vi "Testing.vi"() -> ()   [LabVIEW 2025]
uses:
  <vilib>/measure/madcrms.llb/Basic Averaged DC-RMS for N Chan.vi
  <vilib>/measure/NI_MAPro.lvlib
panel:
  out "Mains Request":sgl
  out "Loop":i32
  out "Bus Current Load Demand":dbl
  out "Bus Voltage RMS/100":dbl
  out "Bus Current Demand to SM":dynamicdata(graph)
  out "All Output Graphs":dynamicdata(graph)
  out "Battery Charge Sw":bool
  out "Battery Discharge Sw":bool
  out "LoadSw3":bool
  out "LoadSw2":bool
  out "LoadSw1":bool
  out "SM PV Current":dbl
  out "SM Wind Current":dbl
  in  "Manual Control\nPV % of Max.":dbl(knob) scale=0.0..100.0
  in  "Manual Control\nWind % of Max.":dbl(knob) scale=0.0..100.0
  in  "Load 3":bool
  in  "Load 2":bool
  in  "Load 1":bool
  out "Bus Current (rms)":dynamicdata(graph)
  out "Bus Voltage (rms)":dynamicdata(graph)
  out "Load 3":bool
  out "Load 2":bool
  out "Load 1":bool
  out "Charge Batt":bool
  out "Discharge Batt":bool
  out "Analog Input (Main Capacity 0-10V)":dynamicdata(graph)
  in  "stop":bool
  out "Voltage Dip Supply < Demand":dynamicdata(graph)
  out "240 Vrms Supply >=Demand":dynamicdata(graph)
  out "Capacity - Demand (current)":dynamicdata(graph)
  in  "Battery Charging Current":dbl
  in  "Battery Disharging Current":dbl
  in  "Load 3 Demand (current)":dbl
  in  "Load 2 Demand (current)":dbl
  in  "Load 1 Demand (current)":dbl
  out "Battery Charging Current":dynamicdata(graph)
  out "Load 3 Current":dynamicdata(graph)
  out "Load 2 Current":dynamicdata(graph)
  out "Load 1 Current":dynamicdata(graph)
  out "Battery Discharging Current (A rms)":dynamicdata(graph)
  out "Main Available Current (A rms)":dynamicdata(graph)
  out "PV Available Current (A rms)":dynamicdata(graph)
  out "Wind Available Current (A rms)":dynamicdata(graph)
  in  "Main capacity (current)":dbl
  in  "Max PV capacity (current)":dbl
  in  "Max wind capacity (current)":dbl
  out "Bus Voltage 240Vrms/100":dynamicdata(graph)
  # "Smart Meter Emulator Algorithm inputs and output status"
  # "Manual testing of Wind/PV inputs and Load calls without using the test bed  - Output graph on right - by Russel Torah - 2021"
  # "Manual Control of Load selection \nPress Load button to activate"
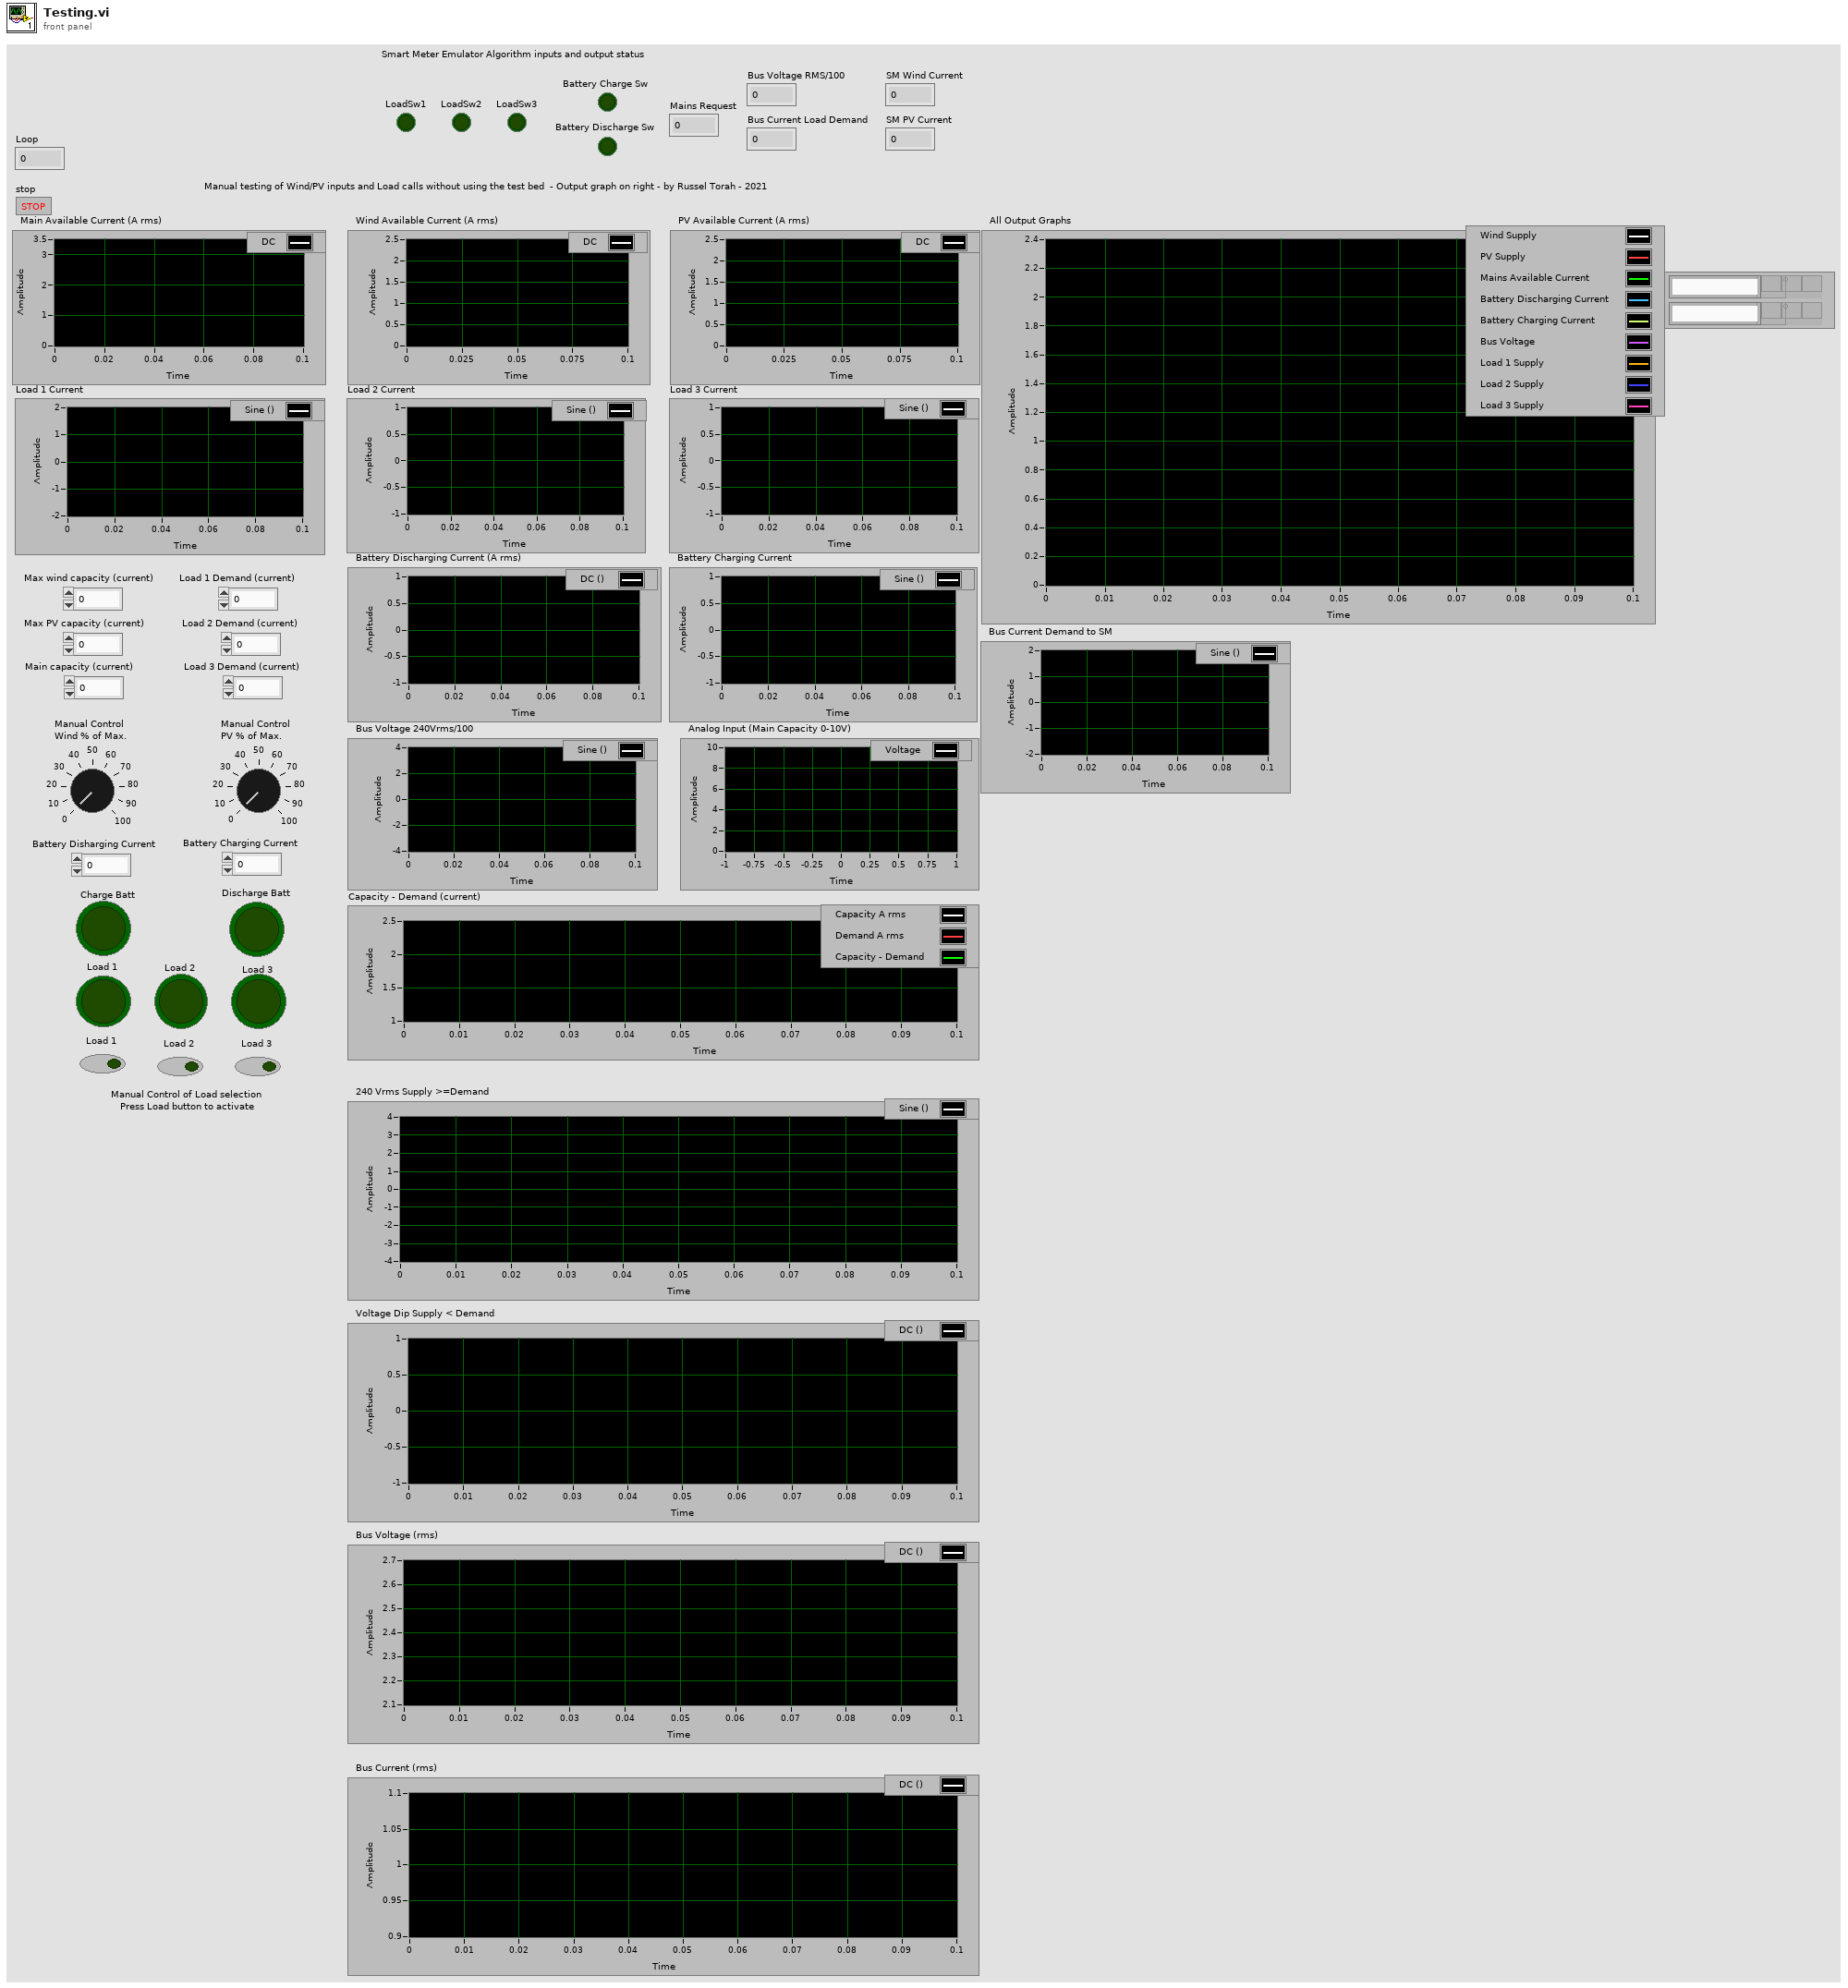
[diagram p1: front panel]
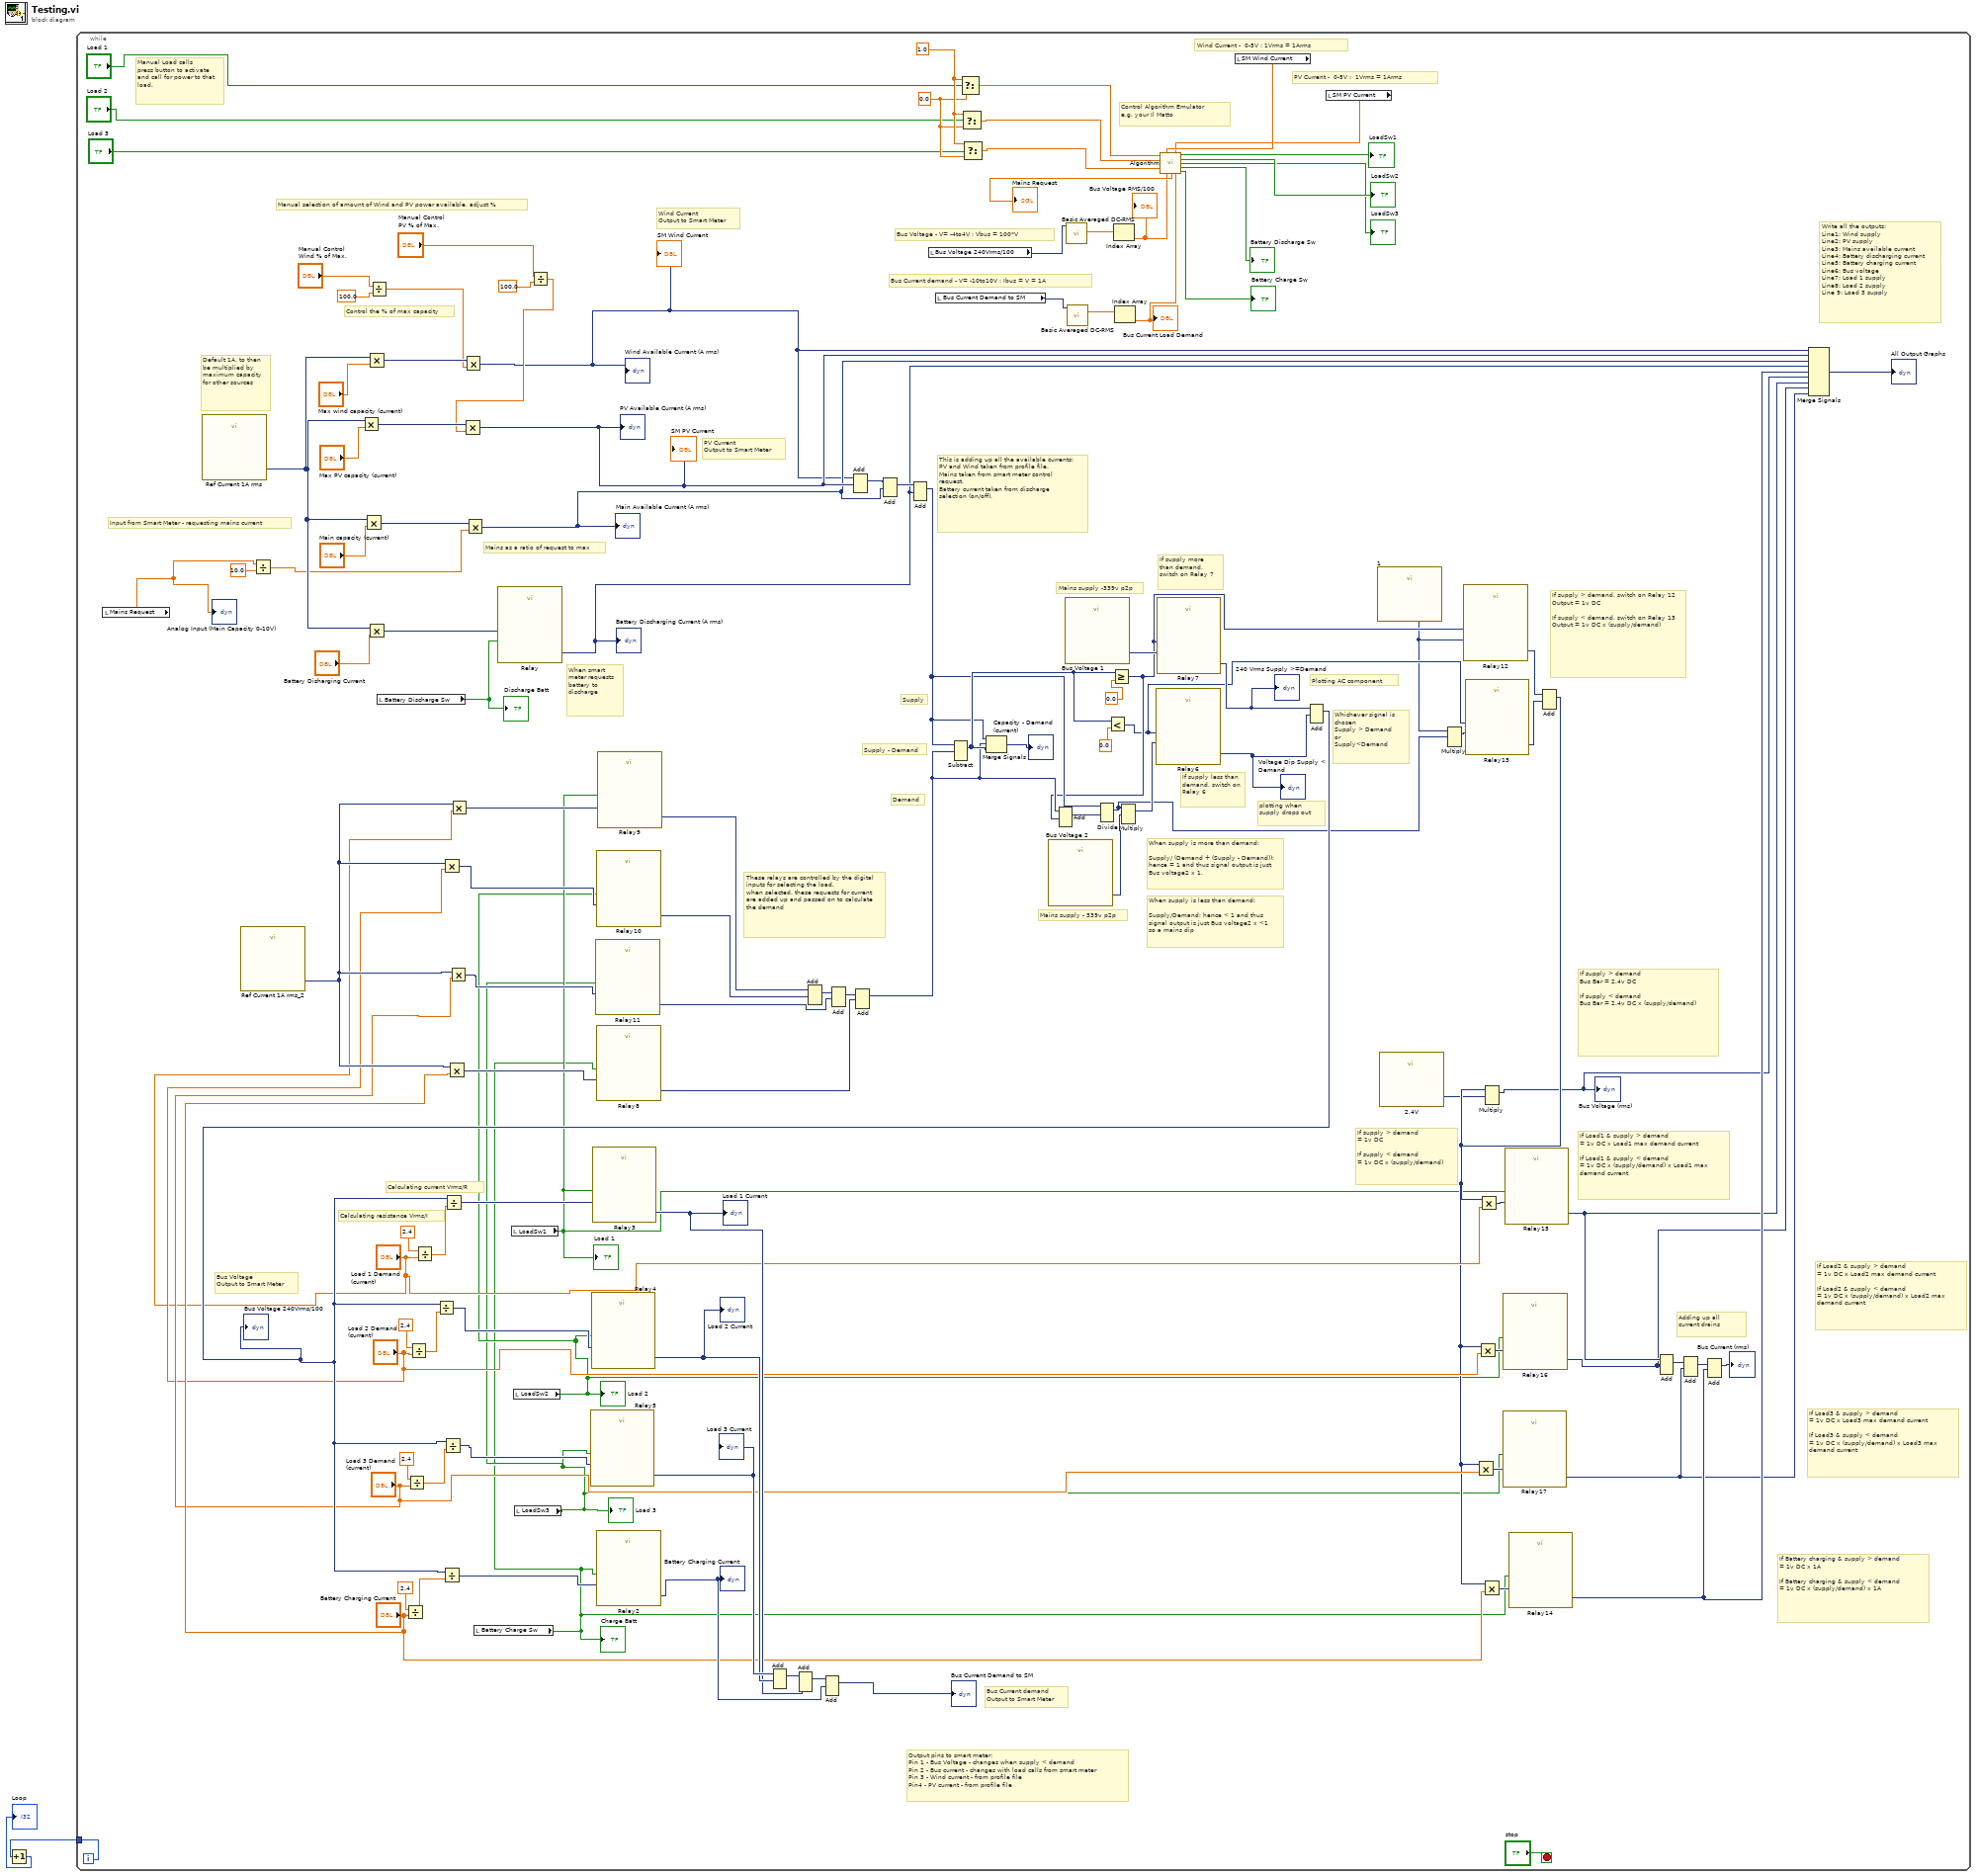
[diagram p0: block diagram]
diagram:
  n1 = while {
    tunnel: [w3] -> w2
    i -> [w3]
    stop <- "stop" stop-if-true
    w32 = 0.0 ("f")
    w33 = 1.0 ("t")
    # "Bus Current demand - V= -10to10V : Ibus = V = 1A"
    # "Bus Voltage - V= -4to4V : Vbus = 100*V"
    # "Wind Current -  0-5V : 1Vrms = 1Arms"
    # "PV Current -  0-5V :  1Vrms = 1Arms"
    # "PV Current\nOutput to Smart Meter"
    # "Wind Current\nOutput to Smart Meter"
    # "Bus Current demand\nOutput to Smart Meter"
    # "Bus Voltage\nOutput to Smart Meter"
    # "Control Algorithm Emulator\ne.g. your Il Matto"
    # "Control the % of max capacity"
    # "Manual selection of amount of Wind and PV power available, adjust %"
    # "Manual Load calls\npress button to activate and call for power to that load."
    # "Plotting AC component"
    # "plotting when supply drops out"
    # "Output pins to smart meter:\nPin 1 - Bus Voltage - changes when supply < demand\nPin 2 - Bus current - changes with load calls from smart meter\nPin 3 - Wind current - from profile file\nPin4 - PV current - from profile file"
    # "When smart meter requests battery to discharge"
    # "Mains as a ratio of request to max"
    # "Write all the outputs:\nLine1: Wind supply\nLine2: PV supply\nLine3: Mains available current\nLine4: Battery discharging current\nLine5: Battery charging current\nLine6: Bus voltage\nLine7: Load 1 supply\nLine8: Load 2 supply\nLine 9: Load 3 supply"
    # "Adding up all current drains"
    # "If Battery charging & supply > demand\n= 1v DC x 1A\n\nIf Battery charging & supply < demand\n= 1v DC x (supply/demand) x 1A"
    # "If Load3 & supply > demand\n= 1v DC x Load3 max demand current\n\nIf Load3 & supply < demand\n= 1v DC x (supply/demand) x Load3 max demand current"
    # "If Load2 & supply > demand\n= 1v DC x Load2 max demand current\n\nIf Load2 & supply < demand\n= 1v DC x (supply/demand) x Load2 max demand current"
    # "If Load1 & supply > demand\n= 1v DC x Load1 max demand current\n\nIf Load1 & supply < demand\n= 1v DC x (supply/demand) x Load1 max demand current"
    # "If supply > demand\n= 1v DC\n\nIf supply < demand\n= 1v DC x (supply/demand)"
    # "If supply > demand\nBus Bar = 2.4v DC\n\nIf supply < demand\nBus Bar = 2.4v DC x (supply/demand)"
    # "If supply > demand, switch on Relay 12\nOutput = 1v DC\n\nIf supply < demand, switch on Relay 13\nOutput = 1v DC x (supply/demand)"
    # "Whichever signal is chosen\nSupply > Demand\nor\nSupply<Demand"
    # "When supply is less than demand:\n\nSupply/Demand; hence < 1 and thus signal output is just Bus voltage2 x <1 so a mains dip"
    # "When supply is more than demand:\n\nSupply/ (Demand + (Supply - Demand)); hence = 1 and thus signal output is just Bus voltage2 x 1."
    # "Demand"
    # "Supply"
    # "If supply less than demand, switch on Relay 6"
    # "If supply more than demand, switch on Relay 7"
    # "Mains supply - 339v p2p"
    # "Mains supply -339v p2p"
    # "Supply - Demand"
    # "Calculating current Vrms/R"
    # "Calculating resistance Vrms/I"
    # "These relays are controlled by the digital inputs for selecting the load.\nwhen selected, these requests for current are added up and passed on to calculate the demand"
    # "Default 1A, to then be multiplied by maximum capacity for other sources"
    # "Input from Smart Meter - requesting mains current"
    # "This is adding up all the available currents:\nPV and Wind taken from profile file.\nMains taken from smart meter control request.\nBattery current taken from discharge selection (on/off)."
    n2 = local read "Mains Request"() -> (w15:sgl)
    "Analog Input (Main Capacity 0-10V)" <- w15
    n3 = call "Ref Current 1A rms"() -> ("DC"=w113:dynamicdata)  [unwired: 14 in, 1 out]
    n4 = call "Ref Current 1A rms_2"() -> ("DC"=w72:dynamicdata)  [unwired: 14 in, 1 out]
    n5 = Divide(x=w15, y=10.0) -> (x/y=w81:dbl)
    n6 = Multiply(x=w113, y="Max PV capacity (current)") -> (x*y=w122:dynamicdata)
    n7 = Multiply(x=w113, y="Main capacity (current)") -> (x*y=w121:dynamicdata)
    n8 = Multiply(x=w113, y="Max wind capacity (current)") -> (x*y=w123:dynamicdata)
    n9 = Multiply(x=w113, y="Battery Disharging Current") -> (x*y=w120:dynamicdata)
    n10 = Divide(x="Manual Control\nWind % of Max.", y=100.0) -> (x/y=w37:dbl)
    n11 = local read "Battery Discharge Sw"() -> (w11:bool)
    "Discharge Batt" <- w11
    n12 = Divide(x=2.4, y="Battery Charging Current") -> (x/y=w101:dbl)
    n13 = Divide(x=2.4, y="Load 3 Demand (current)") -> (x/y=w103:dbl)
    n14 = Divide(x=2.4, y="Load 2 Demand (current)") -> (x/y=w106:dbl)
    n15 = Divide(x=2.4, y="Load 1 Demand (current)") -> (x/y=w109:dbl)
    n16 = Multiply(x=w72, y="Load 2 Demand (current)") -> (x*y=w96:dynamicdata)
    n17 = Multiply(x=w72, y="Battery Charging Current") -> (x*y=w94:dynamicdata)
    n18 = Multiply(x=w72, y="Load 3 Demand (current)") -> (x*y=w95:dynamicdata)
    n19 = Multiply(x=w72, y="Load 1 Demand (current)") -> (x*y=w97:dynamicdata)
    n20 = Multiply(x=w123, y=w37) -> (x*y=w25:dynamicdata)
    "Wind Available Current (A rms)" <- w25
    "SM Wind Current" <- w25
    n21 = Multiply(x=w121, y=w81) -> (x*y=w66:dynamicdata)
    "Main Available Current (A rms)" <- w66
    n22 = local read "Battery Charge Sw"() -> (w12:bool)
    "Charge Batt" <- w12
    n23 = call "Relay"("Enable"=w11, "Signals"=w120) -> ("Result"=w65:dynamicdata)  [unwired: 8 in, 1 out]
    "Battery Discharging Current (A rms)" <- w65
    n24 = local read "LoadSw1"() -> (w21:bool)
    "Load 1" <- w21
    n25 = local read "LoadSw2"() -> (w14:bool)
    "Load 2" <- w14
    n26 = local read "LoadSw3"() -> (w13:bool)
    "Load 3" <- w13
    n27 = Divide(x="Manual Control\nPV % of Max.", y=100.0) -> (x/y=w34:dbl)
    n28 = Multiply(x=w122, y=w34) -> (x*y=w67:dynamicdata)
    "PV Available Current (A rms)" <- w67
    "SM PV Current" <- w67
    n29 = call "Relay11"("Enable"=w13, "Signals"=w95) -> ("Result"=w91:dynamicdata)  [unwired: 8 in, 1 out]
    n30 = call "Relay10"("Enable"=w14, "Signals"=w96) -> ("Result"=w92:dynamicdata)  [unwired: 8 in, 1 out]
    n31 = call "Relay8"("Enable"=w12, "Signals"=w94) -> ("Result"=w90:dynamicdata)  [unwired: 8 in, 1 out]
    n32 = call "Relay9"("Enable"=w21, "Signals"=w97) -> ("Result"=w93:dynamicdata)  [unwired: 8 in, 1 out]
    n33 = Add(1:w92, 2:w93) -> (0:w116:dynamicdata)  [unwired: 1 in, 1 out]
    n34 = Add(1:w91, 2:w116) -> (0:w115:dynamicdata)  [unwired: 1 in, 1 out]
    n35 = Add(1:w67, 2:w25) -> (0:w118:dynamicdata)  [unwired: 1 in, 1 out]
    n36 = Add(1:w90, 2:w115) -> (0:w69:dynamicdata)  [unwired: 1 in, 1 out]
    n37 = Add(1:w66, 2:w118) -> (0:w117:dynamicdata)  [unwired: 1 in, 1 out]
    n38 = Add(1:w65, 2:w117) -> (0:w70:dynamicdata)  [unwired: 1 in, 1 out]
    n39 = local read "Bus Voltage 240Vrms/100"() -> (w8:dynamicdata)
    n40 = local read "Bus Current Demand to SM"() -> (w6:dynamicdata)
    n41 = Subtract(1:w69, 2:w70) -> (0:w71:dynamicdata)  [unwired: 1 in, 1 out]
    n42 = Select(t=w33, s="Load 1", f=w32) -> (s? t:f=w31:dbl)
    n43 = Select(t=w33, s="Load 2", f=w32) -> (s? t:f=w30:dbl)
    n44 = Select(t=w33, s="Load 3", f=w32) -> (s? t:f=w29:dbl)
    n45 = Merge Signals(w70, w69, w71) -> (→"Capacity - Demand (current)":dynamicdata)
    n46 = call "Bus Voltage 2"() -> ("Sine"=w98:dynamicdata)  [unwired: 14 in, 1 out]
    n47 = call "Bus Voltage 1"() -> ("Sine"=w89:dynamicdata)  [unwired: 14 in, 1 out]
    n48 = call-poly <vilib>:"Basic Averaged DC-RMS.vi"("signals in"=w8) -> ("RMS values"=w9:dbl[])  [unwired: 7 in, 3 out]
    n49 = call-poly <vilib>:"Basic Averaged DC-RMS.vi"("signals in"=w6) -> ("RMS values"=w7:dbl[])  [unwired: 7 in, 3 out]
    n50 = Less?(x=w71, y=0.0) -> (x < y?=w63:dynamicdata)
    n51 = Greater Or Equal?(x=w71, y=0.0) -> (x >= y?=w64:dynamicdata)
    n52 = Add(1:w64, 2:w69) -> (0:w86:dynamicdata)  [unwired: 1 in, 1 out]
    n53 = Divide(1:w86, 2:w70) -> (0:w60:dynamicdata)  [unwired: 1 in, 1 out]
    n54 = Index Array(array=w9) -> (element=w5:dbl)  [unwired: 1 in]
    "Bus Voltage RMS/100" <- w5
    n55 = Index Array(array=w7) -> (element=w4:dbl)  [unwired: 1 in]
    "Bus Current Load Demand" <- w4
    n56 = Multiply(1:w98, 2:w60) -> (0:w88:dynamicdata)  [unwired: 1 in, 1 out]
    n57 = call "Relay6"("Enable"=w63, "Signals"=w88) -> ("Result"=w87:dynamicdata)  [unwired: 8 in, 1 out]
    "Voltage Dip Supply < Demand" <- w87
    n58 = call "Relay7"("Enable"=w64, "Signals"=w89) -> ("Result"=w85:dynamicdata)  [unwired: 8 in, 1 out]
    "240 Vrms Supply >=Demand" <- w85
    n59 = local read "SM Wind Current"() -> (w24:dbl)
    n60 = Add(1:w87, 2:w85) -> (0:w83:dynamicdata)  [unwired: 1 in, 1 out]
    "Bus Voltage 240Vrms/100" <- w83
    n61 = Divide(x=w83, y=w106) -> (x/y=w108:dynamicdata)
    n62 = Divide(x=w83, y=w101) -> (x/y=w102:dynamicdata)
    n63 = Divide(x=w83, y=w103) -> (x/y=w105:dynamicdata)
    n64 = Divide(x=w83, y=w109) -> (x/y=w111:dynamicdata)
    n65 = call "Relay5"("Enable"=w13, "Signals"=w105) -> ("Result"=w79:dynamicdata)  [unwired: 8 in, 1 out]
    "Load 3 Current" <- w79
    n66 = call "Relay4"("Enable"=w14, "Signals"=w108) -> ("Result"=w78:dynamicdata)  [unwired: 8 in, 1 out]
    "Load 2 Current" <- w78
    n67 = call "Relay3"("Enable"=w21, "Signals"=w111) -> ("Result"=w77:dynamicdata)  [unwired: 8 in, 1 out]
    "Load 1 Current" <- w77
    n68 = call "Relay2"("Enable"=w12, "Signals"=w102) -> ("Result"=w75:dynamicdata)  [unwired: 8 in, 1 out]
    "Battery Charging Current" <- w75
    n69 = Add(1:w78, 2:w79) -> (0:w80:dynamicdata)  [unwired: 1 in, 1 out]
    n70 = Add(1:w77, 2:w80) -> (0:w76:dynamicdata)  [unwired: 1 in, 1 out]
    n71 = Add(1:w75, 2:w76) -> (0:→"Bus Current Demand to SM":dynamicdata)  [unwired: 1 in, 1 out]
    n72 = local read "SM PV Current"() -> (w23:dbl)
    n73 = call "Algorithm.vi"("LoadCall1"=w31, "Wind available: 0 to 5 V DC"=w24, "PV available: 0 to 5 V DC"=w23, "LoadCall2"=w30, "LoadCall3"=w29, "Bus Voltage IN: -4 to 4 Vrms AC"=w5, "Bus Current IN: -10 to 10 Vrms AC"=w4) -> ("LoadSw1"=→"LoadSw1":bool, "LoadSw2"=→"LoadSw2":bool, "LoadSw3"=→"LoadSw3":bool, "Battery Discharge Sw"=→"Battery Discharge Sw":bool, "Mains Request"=→"Mains Request":sgl, "Battery Charge Sw"=→"Battery Charge Sw":bool)  [unwired: 3 in]
    n74 = call "1"() -> ("DC"=w61:dynamicdata)  [unwired: 14 in, 1 out]
    n75 = call "2.4V"() -> ("DC"=w48:dynamicdata)  [unwired: 14 in, 1 out]
    n76 = Multiply(1:w60, 2:w61) -> (0:w62:dynamicdata)  [unwired: 1 in, 1 out]
    n77 = call "Relay12"("Enable"=w64, "Signals"=w61) -> ("Result"=w59:dynamicdata)  [unwired: 8 in, 1 out]
    n78 = call "Relay13"("Enable"=w63, "Signals"=w62) -> ("Result"=w58:dynamicdata)  [unwired: 8 in, 1 out]
    n79 = Add(1:w58, 2:w59) -> (0:w49:dynamicdata)  [unwired: 1 in, 1 out]
    n80 = Multiply(x=w49, y="Load 3 Demand (current)") -> (x*y=w56:dynamicdata)
    n81 = Multiply(x=w49, y="Load 2 Demand (current)") -> (x*y=w55:dynamicdata)
    n82 = Multiply(x=w49, y="Load 1 Demand (current)") -> (x*y=w54:dynamicdata)
    n83 = Multiply(1:w48, 2:w49) -> (0:w43:dynamicdata)  [unwired: 1 in, 1 out]
    "Bus Voltage (rms)" <- w43
    n84 = Multiply(x=w49, y="Battery Charging Current") -> (x*y=w57:dynamicdata)
    n85 = call "Relay17"("Enable"=w13, "Signals"=w56) -> ("Result"=w40:dynamicdata)  [unwired: 8 in, 1 out]
    n86 = call "Relay16"("Enable"=w14, "Signals"=w55) -> ("Result"=w41:dynamicdata)  [unwired: 8 in, 1 out]
    n87 = call "Relay15"("Enable"=w21, "Signals"=w54) -> ("Result"=w42:dynamicdata)  [unwired: 8 in, 1 out]
    n88 = call "Relay14"("Enable"=w12, "Signals"=w57) -> ("Result"=w44:dynamicdata)  [unwired: 8 in, 1 out]
    n89 = Add(1:w41, 2:w42) -> (0:w47:dynamicdata)  [unwired: 1 in, 1 out]
    n90 = Add(1:w40, 2:w47) -> (0:w46:dynamicdata)  [unwired: 1 in, 1 out]
    n91 = Add(1:w44, 2:w46) -> (0:→"Bus Current (rms)":dynamicdata)  [unwired: 1 in, 1 out]
    n92 = Merge Signals(w25, w67, w66, w65, w44, w43, w42, w41, w40) -> (→"All Output Graphs":dynamicdata)
  }
  n93 = Increment(x=w2) -> (x+1=→"Loop":i32)
